vi "App - analyze RUS V6.vi"() -> ()   [LabVIEW 2018] (continued)
          tunnel: w1620 -> [w1627 w1636]
          tunnel: [w1626 w1637] -> w1619
          tunnel: [w1625 w1638] -> w1618
          tunnel: [w1624 w1640] -> w1617
          frame False {
            n725 = call <vilib>:"Color to RGB.vi"("Color"=u32 10987431) -> ("Resolved Color"=w1630:u32)  [unwired: 3 out]
            n726 = call <vilib>:"Color to RGB.vi"("Color"=u32 7500402) -> ("Resolved Color"=w1632:u32)  [unwired: 3 out]
            n727 = call <vilib>:"Color to RGB.vi"("Color"=u32 8158332) -> ("Resolved Color"=w1634:u32)  [unwired: 3 out]
            n728 = Bundle By Name(cluster=w1629, "BG Color"=w1630) -> (w1624:T43)
            n729 = Bundle By Name(cluster=w1627, "BG Color"=w1632) -> (w1626:T43)
            n730 = Bundle By Name(cluster=w1628, "BG Color"=w1634) -> (w1625:T43)
          }
          frame True {
            n731 = call <vilib>:"Color to RGB.vi"("Color"=u32 10987431) -> ("Resolved Color"=w1642:u32)  [unwired: 3 out]
            n732 = call <vilib>:"Color to RGB.vi"("Color"=u32 7500402) -> ("Resolved Color"=w1644:u32)  [unwired: 3 out]
            n733 = call <vilib>:"Color to RGB.vi"("Color"=u32 8158332) -> ("Resolved Color"=w1646:u32)  [unwired: 3 out]
            n734 = Bundle By Name(cluster=w1641, "BG Color"=w1642) -> (w1640:T43)
            n735 = Bundle By Name(cluster=w1636, "BG Color"=w1644) -> (w1637:T43)
            n736 = Bundle By Name(cluster=w1639, "BG Color"=w1646) -> (w1638:T43)
          }
        }
        n737 = property on="Tab : everything" class="TabCtl (strict)"("Colors"=w1617) -> ()  [unwired: 2 in, 2 out]
        n738 = property on="Tab :  Fit controls" class="TabCtl (strict)"("Colors"=w1618) -> ()  [unwired: 2 in, 2 out]
        n739 = property on="Tab : temperature folder" class="TabCtl (strict)"("Colors"=w1619) -> ()  [unwired: 2 in, 2 out]
      }
      event "Plot: All": Cursor Move {
        n740 = event-data() -> ("CursIdx"=w1650:i32)  [unwired: 1 in]
        n741 = case shown="3..5, Default" w1650 {
          selector: w1650 -> [w1653 w1656]
          tunnel: w1649 -> [w1652 _]
          tunnel: w1648 -> [_ w1655]
          frame 3..5, Default {
            # "zoom cursor bracket"
            n742 = call "cursor window logic V2.vi"("CursIdx"=w1653, "cursor window action"=cursor_window_action."cursor moves", "cursor window in"=w1652) -> ()  [unwired: 7 in, 2 out]
          }
          frame 0..2 {
            # "window  cursor bracket"
            n743 = call "cursor window logic V2.vi"("CursIdx"=w1656, "cursor window action"=cursor_window_action."cursor moves", "cursor window in"=w1655) -> ()  [unwired: 7 in, 2 out]
          }
        }
      }
      event User Event {
        n744 = event-data() -> ("talk to the first loop"=w1666:string)  [unwired: 1 in]
        n745 = call "slide controller.vi"("slide action"=slide_action."check", "slide control"=w1657) -> ("in slide"=w1658:bool)  [unwired: 6 in, 3 out]
        n746 = case shown="\"calculation finished\"" w1666 {
          tunnel: w1665 -> [_ _ w1688]
          tunnel: w1664 -> [_ _ w1687]
          tunnel: w1663 -> [_ w1677 _]
          tunnel: w1662 -> [_ w1675 _]
          tunnel: w1661 -> [_ w1674 _]
          tunnel: w1658 -> [_ _ w1686]
          tunnel: "plot fit progress?" -> [_ _ w1685]
          tunnel: w1657 -> [_ _ w1684]
          frame "False", Default {
          }
          frame "check fragment zoom" {
            n747 = property class="XYGraph (strict)"(reference=w1674) -> ("XScale.Maximum"=w1669:dbl, "XScale.Minimum"=w1668:dbl)  [unwired: 1 in, 2 out]
            n748 = Unbundle By Name(w1675) -> ("f (Hz)"=w1670:dbl)
            n749 = call "Q -- check range.vi"("upper"=w1669, "lower"=w1668, "number"=w1670) -> ("in range?"=w1673:bool)  [unwired: 4 in, 4 out]
            n750 = call "Q - not nan and not zero.vi"("Numeric"=w1670) -> ("Boolean"=w1671:bool)  [unwired: 10 in]
            n751 = Not(x=w1673) -> (.not. x?=w1672:bool)
            n752 = And(x=w1671, y=w1672) -> (x .and. y?=w1667:bool)
            n753 = case shown="\"when out of win\"" "zoom mode" {
              tunnel: w1677 -> [_ w1679 w1682]
              tunnel: w1667 -> [_ w1678 _]
              frame "manual", Default {
              }
              frame "when out of win" {
                n754 = case shown="False" w1678 {
                  tunnel: w1679 -> [_ w1681]
                  frame False {
                  }
                  frame True {
                    w1680 = "scale:frequency window"  # autoscale
                    n755 = Generate User Event(user event=w1681, event data cluster=w1680) -> ()  [unwired: 2 in, 2 out]
                  }
                }
              }
              frame "always" {
                w1683 = "scale:frequency window"  # autoscale
                n756 = Generate User Event(user event=w1682, event data cluster=w1683) -> ()  [unwired: 2 in, 2 out]
              }
            }
          }
          frame "calculation finished" {
            n757 = flat-sequence {
              tunnel: w1687 -> [w1694]
              tunnel: w1686 -> [w1691]
              tunnel: w1685 -> [w1693]
              tunnel: w1688 -> [w1705]
              tunnel: w1684 -> [w1698]
              frame #0 {
                n758 = Not(x=w1693) -> (.not. x?=w1692:bool)
                n759 = And(x=w1692, y=w1691) -> (x .and. y?=w1690:bool)
                n760 = Not(x=w1690) -> (.not. x?=w1689:bool)
                n761 = case shown="True" w1689 {
                  tunnel: w1694 -> [_ w1696]
                  frame False {
                  }
                  frame True {
                    (unwired) 0.0
                    n762 = Generate User Event(user event=w1696, event data cluster="redraw:all" ("event data")) -> ()  [unwired: 2 in, 2 out]
                  }
                }
              }
              frame #1 {
                w1701 = 10  # n
                # "recursively call itself while \"in slide\" is true"
                n763 = local read "in sweep folder"() -> (w1706:bool)
                n764 = call "slide controller.vi"("slide action"=slide_action."check", "slide control"=w1698) -> ("slide control OUT"=w1697:refnum<vi>, "halt event"=w1699:bool)  [unwired: 6 in, 2 out]
                n765 = And(x=w1706, y=w1699) -> (x .and. y?=w1704:bool)
                n766 = case shown="False" w1704 {
                  tunnel: w1705 -> [_ w1709]
                  tunnel: w1697 -> [w1707 _]
                  frame False {
                    n767 = call "slide controller.vi"("slide action"=slide_action."halt", "slide control"=w1707) -> ()  [unwired: 6 in, 4 out]
                  }
                  frame True {
                    w1710 = "next"  # next temperature
                    n768 = Generate User Event(user event=w1709, event data cluster=w1710) -> ()  [unwired: 2 in, 2 out]
                  }
                }
                n769 = Not(x=w1704) -> (.not. x?=w1703:bool)
                n770 = call "mean time interval.vi"("init"=w1703, "n"=w1701) -> ("mean"=→"ms/point":dbl)  [unwired: 8 in, 1 out]
              }
            }
          }
        }
      }
      event User Event {
        n771 = event-data() -> ("autoscale"=w1718:string)  [unwired: 1 in]
        n772 = local read "temperature points"() -> (w1717:dbl[])
        n773 = local read "time points"() -> (w1716:dbl[])
        n774 = case shown="\"scale:freq&atten\"" w1718 {
          tunnel: w1717 -> [_ _ _ _ w1772 _]
          tunnel: w1716 -> [_ _ _ _ _ w1773]
          tunnel: w1713 -> [w1722 _ _ _ _ _]
          tunnel: w1714 -> [w1721 _ _ _ _ _]
          tunnel: w1712 -> [_ _ w1752 _ _ _]
          tunnel: w1715 -> [w1719 _ _ _ _ _]
          tunnel: w1711 -> [_ w1747 _ _ _ _]
          frame "scale:c.plane plot zoom", Default {
            # "false- fixed\ntrue -- zoom"
            n775 = local read "c.plane scale"() -> (w1723:bool)
            n776 = Unbundle By Name(w1719) -> ("4corners.z(inf)"=w1720:cdb)
            n777 = case shown="True" w1723 {
              tunnel: w1722 -> [_ _]
              tunnel: [w1729 w1744] -> w1727
              tunnel: [w1728 w1743] -> w1726
              tunnel: [w1729 w1739] -> w1725
              tunnel: [w1728 w1738] -> w1724
              tunnel: [TRUE FALSE] -> _
              tunnel: w1721 -> [w1732 _]
              tunnel: w1720 -> [_ w1734]
              frame False {
                n778 = Unbundle By Name(w1732) -> ("pond scale factor"=w1731:dbl)
                n779 = Divide(x=w1731, y=2) -> (x/y=w1729:dbl)
                n780 = Negate(x=w1729) -> (-x=w1728:dbl)
              }
              frame True {
                w1736 = cdb 0.0+0.0i  # t
                w1740 = 0.1 ("y")
                n781 = Not A Number/Path/Refnum?(number/path/refnum=w1734) -> (NaN/Path/Refnum?=w1737:bool)
                n782 = Select(t=w1736, s=w1737, f=w1734) -> (s? t:f=w1735:cdb)
                n783 = Complex To Re/Im(x + iy=w1735) -> (x=w1742:dbl, y=w1741:dbl)
                n784 = Subtract(x=w1741, y=w1740) -> (x-y=w1738:dbl)
                n785 = Add(x=w1741, y=w1740) -> (x+y=w1739:dbl)
                n786 = Subtract(x=w1742, y=w1740) -> (x-y=w1743:dbl)
                n787 = Add(x=w1742, y=w1740) -> (x+y=w1744:dbl)
              }
            }
            n788 = property on="Plot: complex plane" class="XYGraph (strict)"("XScale.Maximum"=w1727, "XScale.Minimum"=w1726) -> ()  [unwired: 2 in, 2 out]
            n789 = property on="Plot: complex plane" class="XYGraph (strict)"("YScale.Maximum"=w1725, "YScale.Minimum"=w1724) -> ()  [unwired: 2 in, 2 out]
          }
          frame "rescale All from Zoom cursor" {
            n790 = call "cursor window logic V2.vi"("cursor window action"=cursor_window_action."zoom X", "cursor window in"=w1747) -> ()  [unwired: 8 in, 2 out]
          }
          frame "scale:frequency window" {
            n791 = Unbundle By Name(w1752) -> ("left"=w1759:dbl, "right"=w1758:dbl)
            n792 = Unbundle By Name(w1752) -> ("left"=w1755:dbl, "right"=w1754:dbl)
            n793 = Not A Number/Path/Refnum?(number/path/refnum=w1759) -> (NaN/Path/Refnum?=w1761:bool)
            n794 = Not A Number/Path/Refnum?(number/path/refnum=w1758) -> (NaN/Path/Refnum?=w1760:bool)
            n795 = Not A Number/Path/Refnum?(number/path/refnum=w1755) -> (NaN/Path/Refnum?=w1757:bool)
            n796 = Not A Number/Path/Refnum?(number/path/refnum=w1754) -> (NaN/Path/Refnum?=w1756:bool)
            n797 = Or(x=w1761, y=w1760) -> (x .or. y?=w1751:bool)
            n798 = Or(x=w1757, y=w1756) -> (x .or. y?=w1753:bool)
            n799 = Not(x=w1751) -> (.not. x?=w1750:bool)
            n800 = And(x="freq(T) : auto-adjust Y scale", y=w1750) -> (x .and. y?=w1748:bool)
            n801 = case shown="False" w1753 {
              tunnel: w1755 -> [w1764 _]
              tunnel: w1754 -> [w1763 _]
              frame False {
                n802 = local read "scale gauge: geometry plot"() -> (w1762:dbl)
                n803 = Negate(x=w1762) -> (-x=w1765:dbl)
                n804 = property on="Plot: linear map" class="XYGraph (strict)"("XScale.Minimum"=w1764, "XScale.Maximum"=w1763, "YScale.Maximum"=w1762, "YScale.Minimum"=w1765) -> ()  [unwired: 2 in, 2 out]
                n805 = property on="Plot: fragment" class="XYGraph (strict)"("XScale.Minimum"=w1764, "XScale.Maximum"=w1763) -> ()  [unwired: 2 in, 2 out]
                n806 = property on="Plot: geometry" class="XYGraph (strict)"("YScale.Maximum"=w1762, "YScale.Minimum"=w1765, "XScale.Maximum"=w1762, "XScale.Minimum"=w1765) -> ()  [unwired: 2 in, 2 out]
              }
              frame True {
              }
            }
            n807 = case shown="True" w1748 {
              tunnel: w1759 -> [_ w1767]
              tunnel: w1758 -> [_ w1766]
              frame False {
              }
              frame True {
                n808 = property on="Plot: phase around center" class="XYGraph (strict)"("XScale.Maximum"=w1766, "XScale.Minimum"=w1767) -> ()  [unwired: 2 in, 2 out]
                n809 = property on="Plot: frequency vs T" class="XYGraph (strict)"("YScale.Maximum"=w1766, "YScale.Minimum"=w1767) -> ()  [unwired: 2 in, 2 out]
              }
            }
          }
          frame "scale:freq&atten" {
            n810 = property on="Plot: delta f" class="XYGraph (strict)"() -> ("XScale.Maximum"=w1768:dbl, "XScale.Minimum"=w1769:dbl)  [unwired: 2 in, 2 out]
            n811 = property on="Plot: frequency vs T" class="XYGraph (strict)"("XScale.Maximum"=w1768, "XScale.Minimum"=w1769) -> ()  [unwired: 2 in, 2 out]
            n812 = property on="Plot: attenuation vs T" class="XYGraph (strict)"("XScale.Maximum"=w1768, "XScale.Minimum"=w1769) -> ()  [unwired: 2 in, 2 out]
          }
          frame "scale:temperature" {
            n813 = Array Max & Min(array=w1772) -> (max value=w1771:dbl, min value=w1770:dbl)  [unwired: 2 out]
            n814 = property on="Plot: delta f" class="XYGraph (strict)"("XScale.Maximum"=w1771, "XScale.Minimum"=w1770) -> ()  [unwired: 2 in, 2 out]
            n815 = property on="Plot: frequency vs T" class="XYGraph (strict)"("XScale.Maximum"=w1771, "XScale.Minimum"=w1770) -> ()  [unwired: 2 in, 2 out]
            n816 = property on="Plot: attenuation vs T" class="XYGraph (strict)"("XScale.Maximum"=w1771, "XScale.Minimum"=w1770) -> ()  [unwired: 2 in, 2 out]
          }
          frame "scale:position" {
            n817 = Array Size(array=w1773) -> (size(s)=w1776:i32)
            n818 = Decrement(x=w1776) -> (x-1=w1777:i32)
            n819 = Index Array(array=w1773, index=w1777) -> (element=w1778:dbl)
            n820 = Index Array(array=w1773, index=0) -> (element=w1779:dbl)
            n821 = Max & Min(x=w1778, y=w1779) -> (max(x,y)=w1774:dbl, min(x,y)=w1788:dbl)
            n822 = Add(x=w1788, y=w1774) -> (x+y=w1783:dbl)
            n823 = property on="Plot: Time" class="XYGraph (strict)"("XScale.Maximum"=w1774, "XScale.Minimum"=w1788) -> ()  [unwired: 2 in, 2 out]
            n824 = Divide(x=w1783, y=2.0) -> (x/y=w1785:dbl)
            n825 = property on="Plot: Time" class="XYGraph (strict)"() -> ("CrsrList"=w1780:T44)  [unwired: 2 in, 2 out]
            n826 = call "replace cursor.vi"("action"=enum16{"", "read", "write"}."write" ("Enum"), "cursor index"=0, "new  Y"=0.0, "new X"=w1785, "Cursor List in"=w1780) -> ("Cursor List Out"=w1787:T44)  [unwired: 4 in, 2 out]
            n827 = property on="Plot: Time" class="XYGraph (strict)"("CrsrList"=w1787) -> ()  [unwired: 2 in, 2 out]
          }
        }
      }
      event User Event {
        n828 = event-data() -> ("show plot pallets"=w1789:bool)  [unwired: 1 in]
        n829 = property on="Plot: phase around center" class="XYGraph (strict)"("ScaleLegendVis"=w1789, "Palette Visible"=w1789, "Legend Visible"=w1789) -> ()  [unwired: 2 in, 2 out]
        n830 = property on="Plot: fragment" class="XYGraph (strict)"("ScaleLegendVis"=w1789, "Palette Visible"=w1789, "Legend Visible"=w1789) -> ()  [unwired: 2 in, 2 out]
        n831 = property on="Plot: frequency vs T" class="XYGraph (strict)"("ScaleLegendVis"=w1789, "Palette Visible"=w1789, "Legend Visible"=w1789) -> ()  [unwired: 2 in, 2 out]
        n832 = property on="Plot: attenuation vs T" class="XYGraph (strict)"("ScaleLegendVis"=w1789, "Palette Visible"=w1789, "Legend Visible"=w1789) -> ()  [unwired: 2 in, 2 out]
        n833 = property on="Plot: delta f" class="XYGraph (strict)"("ScaleLegendVis"=w1789, "Palette Visible"=w1789, "Legend Visible"=w1789) -> ()  [unwired: 2 in, 2 out]
        n834 = property on="Plot: All" class="XYGraph (strict)"("ScaleLegendVis"=w1789, "Palette Visible"=w1789, "Legend Visible"=w1789) -> ()  [unwired: 2 in, 2 out]
        n835 = property on="Plot: geometry" class="XYGraph (strict)"("ScaleLegendVis"=w1789, "Palette Visible"=w1789, "Legend Visible"=w1789) -> ()  [unwired: 2 in, 2 out]
        n836 = property on="Plot: linear map" class="XYGraph (strict)"("ScaleLegendVis"=w1789, "Palette Visible"=w1789, "Legend Visible"=w1789) -> ()  [unwired: 2 in, 2 out]
        n837 = property on="Plot: Time" class="XYGraph (strict)"("ScaleLegendVis"=w1789, "Palette Visible"=w1789, "Legend Visible"=w1789) -> ()  [unwired: 2 in, 2 out]
      }
      event User Event {
        n838 = event-data() -> ("redraw"=w1826:string)  [unwired: 1 in]
        n839 = local read "temperature points"() -> (w1823:dbl[])
        n840 = local read "frequency points"() -> (w1825:dbl[])
        n841 = local read "attenuation points"() -> (w1824:dbl[])
        n842 = local read "time points"() -> (w1820:dbl[])
        n843 = local read "time (min)"() -> (w1822:dbl)
        n844 = local read "Magn Field points"() -> (w1792:dbl[])
        n845 = local read "phase points"() -> (w1821:dbl[])
        n846 = local read "power points"() -> (w1794:dbl[])
        n847 = local read "ampl points"() -> (w1804:dbl[])
        n848 = control-ref of="Plot: complex plane"() -> (w1812:refnum<vi>)
        n849 = local read "fit using"() -> (w1806:T5)
        n850 = call "slide controller.vi"("slide action"=slide_action."check", "slide control"=w1798) -> ("in slide"=w1799:bool)  [unwired: 6 in, 3 out]
        n851 = case shown="\"redraw:freq/atten\"" w1826 {
          selector: w1826 -> [_ _ _ _ _ _ w1979 _ _ _]
          tunnel: w1827 -> [_ _ _ w1918 w1929 _ _ _ _ _]
          tunnel: w1816 -> [_ w1890 _ _ _ _ _ _ _ _]
          tunnel: w1817 -> [_ _ _ _ _ _ w1978 w2048 w2058 w2075]
          tunnel: w1814 -> [_ _ _ w1920 _ _ _ _ _ _]
          tunnel: w1818 -> [_ w1885 _ _ _ w1951 _ _ _ _]
          tunnel: w1815 -> [_ w1888 _ _ _ _ _ _ _ _]
          tunnel: w1813 -> [_ w1887 _ _ _ _ _ _ _ _]
          tunnel: w1819 -> [_ w1886 _ _ _ w1950 _ _ _ _]
          tunnel: w1825 -> [_ _ _ _ _ _ w1977 _ w2068 w2076]
          tunnel: w1824 -> [_ _ _ _ _ _ w1976 _ _ w2071]
          tunnel: w1823 -> [_ _ _ _ _ _ w1975 w2032 w2062 _]
          tunnel: w1822 -> [_ _ _ _ _ _ w1974 w2047 _ _]
          tunnel: w1821 -> [_ _ _ _ _ _ w1973 _ _ _]
          tunnel: w1820 -> [_ _ _ _ _ _ w1972 w2029 _ _]
          tunnel: w1809 -> [_ _ _ _ _ _ w1971 _ _ _]
          tunnel: w1793 -> [_ _ _ _ _ _ w1970 _ _ _]
          tunnel: w1812 -> [_ w1884 _ _ _ _ _ _ _ _]
          tunnel: "plot when in slide" -> [_ _ _ _ _ _ w1967 _ _ _]
          tunnel: w1799 -> [_ _ _ _ _ _ w1965 _ _ _]
          tunnel: w1810 -> [_ _ _ _ _ _ w1963 _ w2061 _]
          tunnel: w1808 -> [_ _ _ _ _ _ w1962 _ _ _]
          tunnel: w1807 -> [_ _ _ _ _ _ w1961 _ w2060 _]
          tunnel: w1806 -> [_ _ _ _ _ _ w1960 _ _ _]
          tunnel: w1805 -> [_ _ _ _ _ _ w1959 w2039 _ _]
          tunnel: w1804 -> [_ _ _ _ _ _ w1958 _ _ _]
          tunnel: w1803 -> [_ _ _ _ _ _ w1957 _ _ _]
          tunnel: w1802 -> [_ _ _ _ _ _ w1956 _ _ _]
          tunnel: w1801 -> [_ _ _ _ _ w1936 _ _ _ _]
          tunnel: w1797 -> [_ _ _ _ _ _ w1955 _ _ _]
          tunnel: w1796 -> [_ _ _ _ _ _ w1954 _ _ _]
          tunnel: w1795 -> [_ _ _ _ _ _ w1953 _ _ _]
          tunnel: w1794 -> [_ _ _ _ _ _ w1952 _ _ _]
          tunnel: w1792 -> [_ _ _ _ _ _ _ w2028 _ w2072]
          tunnel: w1791 -> [_ _ _ _ _ _ _ _ _ w2070]
          tunnel: w1790 -> [_ _ _ _ _ _ _ _ _ w2069]
          frame "False", Default {
          }
          frame "redraw:fit related" {
            w1841 = 0.5
            (unwired) FALSE
            # "cursor 1 follows z(inf)\ncursor  2 follows z(0)"
            n852 = Unbundle By Name(w1886) -> ("4corners"=w1889:T12)
            n853 = Unbundle By Name(w1885) -> ("omega in window"=w1865:dbl[], "phase around center"=w1872:dbl[], "three points"=w1863:cluster{dbl[], dbl[]}, "inverse"=w1876:cdb[], "linear"=w1875:cdb[], "omega around"=w1874:dbl[])
            n854 = Unbundle By Name(w1889) -> ("z center"=w1830:cdb, "z(inf)"=w1831:cdb)
            n855 = Unbundle By Name(w1885) -> ("normalized z"=w1835:cdb[], "number of 2D grid points"=w1828:i32)
            n856 = Unbundle By Name(w1888) -> ("wave number"=w1837:dbl)
            n857 = Unbundle By Name(w1889) -> ("z center"=w1829:cdb, "z(0)"=w1844:cdb)
            n858 = Unbundle By Name(w1887) -> ("delta  z"=w1838:cdb)
            n859 = Unbundle By Name(w1890) -> ("omega"=w1869:dbl, "gamma"=w1868:dbl, "theta0"=w1867:dbl)
            n860 = Build Array(w1869, w1868, w1867) -> (w1866:dbl[])
            n861 = Complex To Re/Im(x + iy=w1838) -> (x=w1839:dbl)  [unwired: 1 out]
            n862 = Complex To Re/Im(x + iy=w1831) -> (x=w1857:dbl, y=w1856:dbl)
            n863 = flat-sequence {
              tunnel: w1886 -> [w1910]
              tunnel: w1889 -> [w1909]
              tunnel: w1874 -> [w1898]
              tunnel: [w1897] -> w1873
              frame #0 {
                n864 = Unbundle By Name(w1909) -> ("z center"=w1908:cdb, "z(inf)"=w1906:cdb)
                n865 = Unbundle By Name(w1910) -> ("f (Hz)"=w1904:dbl, "G (Hz)"=w1902:dbl)
                n866 = Subtract(x=w1908, y=w1906) -> (x-y=w1907:cdb)
                n867 = Subtract(x=w1898, y=w1904) -> (x-y=w1903:dbl[])
                n868 = Multiply(x=w1907, y=cdb 2.0+0.0i) -> (x*y=w1894:cdb)
                n869 = Multiply(x=cdb 0.0-1.0i ("y"), y=w1894) -> ()  [unwired: 1 out]
                n870 = Divide(x=w1903, y=w1902) -> (x/y=w1901:dbl[])
                n871 = Add(x=w1894, y=w1906) -> ()  [unwired: 1 out]
                n872 = Multiply(x=w1901, y=2) -> (x*y=w1899:dbl[])
                n873 = Complex To Polar(r * e^(i*theta)=w1894) -> (r=w1893:dbl)  [unwired: 1 out]
                n874 = Negate(x=w1893) -> (-x=w1892:dbl)
                n875 = Multiply(x=w1899, y=w1892) -> (x*y=w1895:dbl[])
                n876 = Bundle("omega around"=w1898, w1895) -> (w1897:cluster{"omega around":dbl[], dbl[]})  [unwired: 1 in]
              }
            }
            n877 = call "omega map fit function.vi"("X"=w1865, "a"=w1866) -> ("f(X,a)"=w1864:dbl[])  [unwired: 2 in, 2 out]
            n878 = call "replace cursor - plot ref.vi"("action"=enum16{"", "read", "write"}."write" ("Enum"), "cursor index"=1, "new  Y"=w1856, "new X"=w1857, "Plot ref in"=w1884) -> ("Plot ref out"=w1836:refnum<vi>)  [unwired: 4 in, 2 out]
            n879 = Divide(x=w1839, y=w1828) -> (x/y=w1840:dbl)
            n880 = Complex To Re/Im(x + iy=w1835) -> (x=w1861:dbl[], y=w1860:dbl[])
            n881 = Divide(x=w1839, y=w1837) -> (x/y=w1849:dbl)
            n882 = Complex To Re/Im(x + iy=w1830) -> (x=w1853:dbl, y=w1852:dbl)
            n883 = Add(x=w1849, y=w1840) -> (x+y=w1848:dbl)
            n884 = Complex To Re/Im(x + iy=w1829) -> (x=w1845:dbl, y=w1846:dbl)
            n885 = Subtract(x=w1844, y=w1829) -> (x-y=w1843:cdb)
            n886 = Bundle("omega in window"=w1865, "f(X,a)"=w1864) -> (w1862:cluster{"omega in window":dbl[], "f(X,a)":dbl[]})  [unwired: 1 in]
            n887 = Bundle("omega in window"=w1865, "phase around center"=w1872) -> (w1871:T45)  [unwired: 1 in]
            n888 = Bundle(w1861, w1860) -> (w1891:cluster{dbl[], dbl[]})  [unwired: 1 in]
            n889 = Complex To Polar(r * e^(i*theta)=w1843) -> (theta=w1842:dbl)  [unwired: 1 out]
            n890 = call "replace cursor - plot ref.vi"("action"=enum16{"", "read", "write"}."write" ("Enum"), "cursor index"=2, "new  Y"=w1852, "new X"=w1853, "Plot ref in"=w1836) -> ()  [unwired: 4 in, 3 out]
            n891 = Build Array(w1871, w1863, w1862) -> (→"Plot: phase around center":T46)
            n892 = call "draw a circle.vi"("angular arc bounds"=w1841, "angular arc center"=w1842, "center Y"=w1846, "center x"=w1845, "radius"=w1849) -> ("output cluster"=w1850:cluster{dbl[], dbl[]})  [unwired: 6 in]
            n893 = call "draw a circle.vi"("angular arc bounds"=w1841, "angular arc center"=w1842, "center Y"=w1846, "center x"=w1845, "radius"=w1848) -> ("output cluster"=w1847:cluster{dbl[], dbl[]})  [unwired: 6 in]
            n894 = Complex To Re/Im(x + iy=w1875) -> (x=w1879:dbl[])  [unwired: 1 out]
            n895 = Complex To Re/Im(x + iy=w1876) -> (x=w1882:dbl[], y=w1881:dbl[])
            n896 = call "draw - 4 corner circle.vi"("4corners"=w1889) -> ("line two"=w1832:cluster{dbl[], dbl[]}, "line one"=w1833:cluster{dbl[], dbl[]}, "circle"=w1834:cluster{dbl[], dbl[]})  [unwired: 8 in]
            n897 = Bundle(w1882, w1881) -> (w1880:cluster{dbl[], dbl[]})  [unwired: 1 in]
            n898 = Bundle("omega around"=w1874, w1879) -> (w1878:cluster{"omega around":dbl[], dbl[]})  [unwired: 1 in]
            n899 = Build Array(w1891, w1880) -> (→"Plot: geometry":cluster{dbl[], dbl[]}[])
            n900 = Build Array(w1891, w1834, w1833, w1832, w1850, w1847) -> (→"Plot: complex plane":cluster{dbl[], dbl[]}[])
            n901 = Build Array(w1878, w1873) -> (→"Plot: linear map":cluster{"omega around":dbl[], dbl[]}[])
          }
          frame "plot filter progress" {
            n902 = control-ref of="Tab : fit/filter progress"() -> (w1916:refnum<vi>)
            n903 = local read "plot filter progress?"() -> (w1912:bool)
            n904 = Not(x=w1912) -> (.not. x?=w1911:bool)
            n905 = Select(t=enum32{"Page 1", "Page 2"}."Page 2" ("Value"), s=w1911, f=enum32{"Page 1", "Page 2"}."Page 1" ("Value")) -> (s? t:f=w1915:enum32{"Page 1", "Page 2"})
            n906 = property class="TabCtl (strict)"(reference=w1916, "Value"=w1915) -> ()  [unwired: 1 in, 2 out]
            n907 = local write "plot filter progress?"(w1911) -> ()
          }
          frame "redraw:all" {
            n908 = case shown="True" "old staff plot" {
              tunnel: [w1921 w1923] -> w1919
              tunnel: w1918 -> [w1921 w1922]
              frame False {
              }
              frame True {
                n909 = Generate User Event(user event=w1922, event data cluster="redraw:fit and fragment" ("event data")) -> (user event out=w1923:refnum<user-event>)  [unwired: 2 in, 1 out]
              }
            }
            n910 = case shown="True" w1920 {
              tunnel: w1919 -> [_ w1927]
              frame False {
              }
              frame True {
                n911 = Generate User Event(user event=w1927, event data cluster="redraw:freq/atten" ("event data")) -> (user event out=w1926:refnum<user-event>)  [unwired: 2 in, 1 out]
                n912 = Generate User Event(user event=w1926, event data cluster="redraw:magn field" ("event data")) -> ()  [unwired: 2 in, 2 out]
              }
            }
          }
          frame "redraw:fit and fragment" {
            n913 = Generate User Event(user event=w1929, event data cluster="redraw:fragment" ("event data")) -> (user event out=w1932:refnum<user-event>)  [unwired: 2 in, 1 out]
            n914 = Generate User Event(user event=w1932, event data cluster="redraw:fit related" ("event data")) -> ()  [unwired: 2 in, 2 out]
          }
          frame "redraw:fragment" {
            # "construct Lorentzian"
            n915 = Unbundle By Name(w1951) -> ("omega in window"=w1949:dbl[], "normalized z"=w1948:cdb[])
            n916 = disable-structure shown="Disabled" {
              frame Disabled {
                n917 = local read item#-1() -> ()  [unwired: 1 out]
                n918 = local read item#-1() -> ()  [unwired: 1 out]
              }
              frame Enabled {
              }
            }
            n919 = Unbundle By Name(w1950) -> ("f (Hz)"=w1935:dbl)
            n920 = call "replace cursor - plot ref.vi"("action"=enum16{"", "read", "write"}."write", "cursor index"=3, "new X"=w1935, "Plot ref in"=w1936) -> ()  [unwired: 5 in, 3 out]
            n921 = call "construct lorentzian.vi"("omega  in"=w1949, "lorentzian"=w1950) -> ("omega  out"=w1940:dbl[], "z out"=w1941:cdb[])  [unwired: 8 in]
            n922 = Complex To Re/Im(x + iy=w1948) -> (x=w1945:dbl[], y=w1944:dbl[])
            n923 = Complex To Re/Im(x + iy=w1941) -> (x=w1943:dbl[], y=w1942:dbl[])
            n924 = Bundle("omega in window"=w1949, w1945) -> (w1939:cluster{"omega in window":dbl[], dbl[]})  [unwired: 1 in]
            n925 = Bundle("omega  out"=w1940, w1943) -> (w1947:cluster{"omega  out":dbl[], dbl[]})  [unwired: 1 in]
            n926 = Bundle("omega  out"=w1940, w1942) -> (w1946:cluster{"omega  out":dbl[], dbl[]})  [unwired: 1 in]
            n927 = Bundle("omega in window"=w1949, w1944) -> (w1938:cluster{"omega in window":dbl[], dbl[]})  [unwired: 1 in]
            n928 = Build Array(w1939, w1938, w1947, w1946) -> (→"Plot: fragment":cluster{"omega  out":dbl[], dbl[]}[])
          }
          frame "redraw:freq/atten" {
            n929 = call "counter-i.vi"("init ?"=w1956, "cricket interval"=30 ("interval")) -> ("cricket"=w1968:bool)  [unwired: 8 in, 1 out]
            n930 = Not(x=w1965) -> (.not. x?=w1964:bool)
            n931 = Compound Arithmetic op=OR(w1967, w1968, w1964) -> (w1966:bool)
            n932 = case shown="True" w1966 {
              tunnel: w1979 -> [_ w2000]
              tunnel: w1978 -> [_ w1999]
              tunnel: w1977 -> [_ w1998]
              tunnel: w1976 -> [_ w1997]
              tunnel: w1975 -> [_ w1996]
              tunnel: w1974 -> [_ w1995]
              tunnel: w1973 -> [_ w1994]
              tunnel: w1972 -> [_ w1993]
              tunnel: w1971 -> [_ w1987]
              tunnel: w1970 -> [_ w1992]
              tunnel: w1963 -> [_ w1991]
              tunnel: w1962 -> [_ w1990]
              tunnel: w1961 -> [_ w1989]
              tunnel: w1960 -> [_ w1988]
              tunnel: w1959 -> [_ w1986]
              tunnel: w1958 -> [_ w1985]
              tunnel: w1957 -> [_ w1984]
              tunnel: w1955 -> [_ w1983]
              tunnel: w1954 -> [_ w1982]
              tunnel: w1953 -> [_ w1981]
              tunnel: w1952 -> [_ w1980]
              frame False {
              }
              frame True {
                n933 = flat-sequence {
                  tunnel: w2000 -> [_]
                  tunnel: [w2026] -> _
                  tunnel: w1999 -> [w2010]
                  tunnel: w1998 -> [w2004]
                  tunnel: w1997 -> [w2003]
                  tunnel: w1996 -> [w2013]
                  tunnel: w1995 -> [w2025]
                  tunnel: w1994 -> [_]
                  tunnel: w1993 -> [w2018]
                  tunnel: w1987 -> [w2019]
                  tunnel: w1992 -> [w2024]
                  tunnel: w1991 -> [_]
                  tunnel: w1990 -> [w2021]
                  tunnel: w1989 -> [w2020]
                  tunnel: w1988 -> [w2016]
                  tunnel: w1986 -> [_]
                  tunnel: [w2019] -> _
                  tunnel: w1985 -> [_]
                  tunnel: w1984 -> [_]
                  tunnel: w1983 -> [w2012]
                  tunnel: w1982 -> [w2006]
                  tunnel: w1981 -> [w2005]
                  tunnel: w1980 -> [w2002]
                  frame #0 {
                    w2007 = T3."linear-linear" ("mapping")
                    (unwired) FALSE  # plot phase/ampl
                    (unwired) TRUE
                    # "\"scale:frequency window\""
                    # "current point"
                    n934 = Generate User Event(user event=w2012, event data cluster="scale:freq&atten" ("event data")) -> ()  [unwired: 2 in, 2 out]
                    n935 = call "fit function selector.vi"("fit using"=w2016, "temperature"=w2013) -> ("freq out"=w2014:dbl[])  [unwired: 7 in, 2 out]
                    n936 = Subtract(x=w2004, y=w2014) -> (x-y=w2017:dbl[])
                    "delta-f points" <- w2017
                    n937 = Threshold 1D Array(2:w2025, 3:w2018) -> (0:w2027:dbl)  [unwired: 1 in]
                    n938 = Index Array(array=w2013, index=w2027) -> (element=w2026:dbl)
                    n939 = call "color split.vi"("point style"=enum16{"dot", "cross"}."dot", "mapping"=w2020, "tfolder"=w2010, "Plot Ref"=w2019, "Y"=w2004, "X"=w2013) -> ()  [unwired: 5 in, 1 out]
                    n940 = call "color split.vi"("point style"=enum16{"dot", "cross"}."dot", "mapping"=w2020, "tfolder"=w2010, "Plot Ref"=w2024, "Y"=w2003, "X"=w2013) -> ()  [unwired: 5 in, 1 out]
                    n941 = call "color split.vi"("point style"=enum16{"dot", "cross"}."dot", "mapping"=w2007, "tfolder"=w2010, "Plot Ref"=w2005, "Y"=w2003, "X"=w2002) -> ()  [unwired: 5 in, 1 out]
                    n942 = call "color split.vi"("point style"=enum16{"dot", "cross"}."dot", "mapping"=w2007, "tfolder"=w2010, "Plot Ref"=w2006, "Y"=w2004, "X"=w2002) -> ()  [unwired: 5 in, 1 out]
                    n943 = call "color split.vi"("point style"=enum16{"dot", "cross"}."dot", "mapping"="mapping delta f vs T", "tfolder"=w2010, "Plot Ref"=w2021, "Y"=w2017, "X"=w2013) -> ()  [unwired: 5 in, 1 out]
                  }
                }
              }
            }
          }
          frame "redraw:time" {
            w2036 = FALSE  # Name Visible
            # "current point"
            n944 = Threshold 1D Array(2:w2047, 3:w2029) -> (0:w2046:dbl)  [unwired: 1 in]
            n945 = Index Array(array=w2032, index=w2046) -> (element=w2041:dbl)
            n946 = Index Array(array=w2029, index=w2046) -> (element=w2043:dbl)
            n947 = Build Array(w2043) -> (w2042:dbl[])
            n948 = Build Array(w2041) -> (w2044:dbl[])
            n949 = Bundle(w2042, w2044) -> (w2045:cluster{dbl[], dbl[]})  [unwired: 1 in]
            n950 = Bundle("time points"=w2029, "temperature points"=w2032) -> (w2051:T47)  [unwired: 1 in]
            n951 = Build Array(w2045, w2051) -> (w2040:T48)
            n952 = Array Size(array=w2040) -> (size(s)=w2037:i32)
            n953 = call "derivative.vi"("temperature (min)"=w2029, "frequency (kHz)"=w2032) -> ("derivative (kHz/min)"=w2033:dbl[])  [unwired: 9 in]
            n954 = for {
              N: w2037 -> [_]
              tunnel: w2039 -> [w2057]
              tunnel: [w2056] -> w2038
              i -> [w2055]
              n955 = call "plot -- make visible.vi"("Active Plot"=w2055, "reference"=w2057) -> ("reference out"=w2056:refnum<vi>)  [unwired: 9 in]
            }
            n956 = Bundle("temperature points"=w2032, "derivative (kHz/min)"=w2033) -> (w2035:T49)  [unwired: 1 in]
            n957 = Bundle("time points"=w2029, "Magn Field points"=w2028) -> (w2031:T50)  [unwired: 1 in]
            n958 = call "color split.vi"("point style"=enum16{"dot", "cross"}."cross", "tfolder"=w2048, "Plot Ref"=w2038, "plot array IN"=w2040, "Y"=w2032, "X"=w2029) -> ("plot array OUT"=w2050:T51)  [unwired: 5 in]
            n959 = Build Array(w2035) -> (→"Plot: dTemp/dTime":T52)
            n960 = Build Array(w2031) -> (w2030:T53)
            n961 = Unbundle By Name(w2048) -> ("timestamp array"=w2054:dbl[])
            n962 = local write "Plot: H vs Time"(w2030) -> ()
            n963 = Array Max & Min(array=w2032) -> (max value=w2053:dbl, min value=w2052:dbl)  [unwired: 2 out]
            n964 = call "generate comb.vi"("maxY"=w2053, "Name Visible"=w2036, "minY"=w2052, "Plot Ref"=w2038, "freq array"=w2054, "plot list IN"=w2050) -> ()  [unwired: 5 in, 1 out]
          }
          frame "redraw:dfdt" {
            w2059 = enum16{"dot", "cross"}."dot"  # point style
            n965 = call "derivative d Log f.vi"("log T ?"="log T ?", "requested size"="derivative window", "temperature (min)"=w2062, "frequency (kHz)"=w2068) -> ("derivative (kHz/min)"=w2067:dbl[])  [unwired: 7 in]
            n966 = Multiply(x=w2067, y="zoom factor - derivative") -> (x*y=w2063:dbl[])
            n967 = call "color split.vi"("point style"=w2059, "mapping"=w2060, "tfolder"=w2058, "Plot Ref"=w2061, "Y"=w2063, "X"=w2062) -> ()  [unwired: 5 in, 1 out]
          }
          frame "redraw:magn field" {
            w2073 = T3."linear-linear" ("mapping")
            w2074 = enum16{"dot", "cross"}."dot"  # point style
            n968 = call "color split.vi"("point style"=w2074, "mapping"=w2073, "tfolder"=w2075, "Plot Ref"=w2070, "Y"=w2076, "X"=w2072) -> ()  [unwired: 5 in, 1 out]
            n969 = call "color split.vi"("point style"=w2074, "mapping"=w2073, "tfolder"=w2075, "Plot Ref"=w2069, "Y"=w2071, "X"=w2072) -> ()  [unwired: 5 in, 1 out]
          }
        }
      }
      event User Event {
        n970 = event-data() -> ("cursors"=w2083:string)  [unwired: 1 in]
        n971 = case shown="\"cursors:init all\", Default" w2083 {
          tunnel: cursor_window_action."check" ("cursor window action") -> [_ _ w2137]
          tunnel: w2078 -> [w2085 _ _]
          tunnel: w2079 -> [w2084 _ _]
          tunnel: w2081 -> [w2089 _ w2140]
          tunnel: w2080 -> [w2088 _ w2139]
          tunnel: w2082 -> [w2087 _ w2138]
          frame "cursors:init all", Default {
            w2086 = cursor_window_action."init" ("cursor window action")
            # "init satff"
            n972 = local read "cursor bracket: All, data window"() -> (w2096:T24)
            n973 = Build Array(0, 1, 2) -> (w2106:i32[])
            n974 = local read "cursor bracket: All,  zoom"() -> (w2102:T24)
            n975 = Build Array(3, 4, 5) -> (w2101:i32[])
            n976 = Build Array(0, 1, 2) -> (w2100:i32[])
            n977 = local read "cursor bracket: fragment"() -> (w2098:T24)
            n978 = Bundle By Name(cluster=w2098, "Plot ref"=w2085, "cursors"=w2100) -> (w2099:T24)
            n979 = Bundle By Name(cluster=w2102, "Plot ref"=w2084, "cursors"=w2101) -> (w2103:T24)
            n980 = Bundle By Name(cluster=w2096, "Plot ref"=w2084, "cursors"=w2106) -> (w2097:T24)
            n981 = call "cursor window logic V2.vi"("cursor window action"=w2086, "cursor window in"=w2087, "cursor window init"=w2099) -> ()  [unwired: 7 in, 2 out]
            n982 = call "cursor window logic V2.vi"("cursor window action"=w2086, "cursor window in"=w2088, "cursor window init"=w2103) -> ()  [unwired: 7 in, 2 out]
            n983 = call "cursor window logic V2.vi"("cursor window action"=w2086, "cursor window in"=w2089, "cursor window init"=w2097) -> ()  [unwired: 7 in, 2 out]
          }
          frame "cursor:init colors" {
            w2114 = "zoom:right"  # Name
            w2116 = "zoom:center"  # Name
            w2117 = "zoom:left"  # Name
            w2122 = "win:right"  # Name
            w2124 = "win:center"  # Name
            w2125 = "win:left"  # Name
            w2128 = 0  # index
            w2130 = "win:left"  # Name
            w2136 = u32 0  # Cursor Mode
            w2135 = TRUE  # Allow Drag
            w2134 = FALSE  # Name Visible
            w2133 = u8 0  # Point Style
            w2132 = u8 2  # Style
            w2129 = T44 [{"Name"="win:left", "Color"=16771584, "Style"=2, "Point Style"=0, "Name Visible"=FALSE, "Allow Drag"=TRUE, "Cursor Mode"=0, "Plot"=0, "Index"=0, "Position"={"X"=2535.2200767392833, "Y"=0.0}, "X Scale"=0, "Y Scale"=0, "Watch Plots"=[], "Watch All Plots"=FALSE, "Plot Area"=0, "Label Offset"={"X"=0.6062171324215342, "Y"=9.61538461538465e-05}}, {"Name"="win:center", "Color"=16776960, "Style"=2, "Point Style"=0, "Name Visible"=FALSE, "Allow Drag"=TRUE, "Cursor Mode"=0, "Plot"=0, "Index"=0, "Position"={"X"=2557.3470020726513, "Y"=0.0}, "X Scale"=0, "Y Scale"=0, "Watch Plots"=[], "Watch All Plots"=FALSE, "Plot Area"=0, "Label Offset"={"X"=0.3031085662105397, "Y"=9.61538461538465e-05}}, {"Name"="win:right", "Color"=16771584, "Style"=2, "Point Style"=0, "Name Visible"=FALSE, "Allow Drag"=TRUE, "Cursor Mode"=0, "Plot"=0, "Index"=0, "Position"={"X"=2579.4739274060194, "Y"=0.0}, "X Scale"=0, "Y Scale"=0, "Watch Plots"=[], "Watch All Plots"=FALSE, "Plot Area"=0, "Label Offset"={"X"=0.6062171324210794, "Y"=9.61538461538465e-05}}, {"Name"="zoom:left", "Color"=9013641, "Style"=2, "Point Style"=6, "Name Visible"=FALSE, "Allow Drag"=TRUE, "Cursor Mode"=0, "Plot"=0, "Index"=0, "Position"={"X"=2438.615046565618, "Y"=0.0}, "X Scale"=0, "Y Scale"=0, "Watch Plots"=[], "Watch All Plots"=FALSE, "Plot Area"=0, "Label Offset"={"X"=-0.08660244748853074, "Y"=9.61538461538465e-05}}, {"Name"="zoom:center", "Color"=9013641, "Style"=2, "Point Style"=6, "Name Visible"=FALSE, "Allow Drag"=TRUE, "Cursor Mode"=0, "Plot"=0, "Index"=0, "Position"={"X"=2518.3975513146, "Y"=0.0}, "X Scale"=0, "Y Scale"=0, "Watch Plots"=[], "Watch All Plots"=FALSE, "Plot Area"=0, "Label Offset"={"X"=0.15155428310526986, "Y"=9.61538461538465e-05}}, {"Name"="zoom:right", "Color"=9013641, "Style"=2, "Point Style"=6, "Name Visible"=FALSE, "Allow Drag"=TRUE, "Cursor Mode"=0, "Plot"=0, "Index"=0, "Position"={"X"=2598.1800560635825, "Y"=0.0}, "X Scale"=0, "Y Scale"=0, "Watch Plots"=[], "Watch All Plots"=FALSE, "Plot Area"=0, "Label Offset"={"X"=0.08660244748853074, "Y"=9.61538461538465e-05}}]  # all cursor list
            # "setup cursors"
            n984 = Index Array(array=w2129, index=w2128) -> (element=w2127:T54)
            n985 = Bundle By Name(cluster=w2127, "Name"=w2130, "Color"=u32 16768256, "Style"=w2132, "Point Style"=w2133, "Name Visible"=w2134, "Allow Drag"=w2135, "Cursor Mode"=w2136) -> (w2110:T54)
            n986 = Bundle By Name(cluster=w2110, "Name"=w2117, "Color"=u32 7763574) -> (w2113:T54)
            n987 = Bundle By Name(cluster=w2110, "Name"=w2125, "Color"=u32 13696834) -> (w2121:T54)
            n988 = Bundle By Name(cluster=w2110, "Name"=w2116, "Color"=u32 13816530) -> (w2112:T54)
            n989 = Bundle By Name(cluster=w2110, "Name"=w2114, "Color"=u32 10132122) -> (w2111:T54)
            n990 = Bundle By Name(cluster=w2110, "Name"=w2124, "Color"=u32 16252785) -> (w2120:T54)
            n991 = Bundle By Name(cluster=w2110, "Name"=w2122, "Color"=u32 13959025) -> (w2119:T54)
            n992 = Build Array(w2113, w2112, w2111) -> ()  [unwired: 1 out]
            n993 = Build Array(w2121, w2120, w2119) -> ()  [unwired: 1 out]
          }
          frame "cursors:check all" {
            n994 = call "cursor window logic V2.vi"("cursor window action"=w2137, "cursor window in"=w2138) -> ()  [unwired: 8 in, 2 out]
            n995 = call "cursor window logic V2.vi"("cursor window action"=w2137, "cursor window in"=w2139) -> ()  [unwired: 8 in, 2 out]
            n996 = call "cursor window logic V2.vi"("cursor window action"=w2137, "cursor window in"=w2140) -> ()  [unwired: 8 in, 2 out]
          }
        }
      }
      event "scale gauge: geometry plot": Value Change {
        (unwired) FALSE ("event data")
        n997 = event-data() -> ()  [unwired: 1 in, 1 out]
        n998 = Generate User Event(user event=w2141, event data cluster="scale:frequency window" ("event data")) -> ()  [unwired: 2 in, 2 out]
      }
      event "Plot: Time": Cursor Move {
        n999 = event-data() -> ("CursIdx"=w2145:i32)  [unwired: 1 in]
        n1000 = case shown="1..3" w2145 {
          selector: w2145 -> [w2147 w2159]
          tunnel: w2144 -> [_ w2158]
          tunnel: w2143 -> [w2149 _]
          frame 0, Default {
            w2150 = enum16{"hide", "show x", "show y", "show (x,y)"}."hide"  # label
            w2154 = enum16{"", "read", "write"}."write"  # action
            w2156 = enum16{"", "read", "write"}."read"  # action
            # "green cursor -- current position"
            n1001 = local read "temperature points"() -> (w2155:dbl[])
            n1002 = local read "time points"() -> (w2153:dbl[])
            n1003 = call "replace cursor - plot ref.vi"("action"=w2156, "cursor index"=w2147, "Plot ref in"=w2149) -> ("read X"=w2152:dbl, "Plot ref out"=w2148:refnum<vi>)  [unwired: 6 in, 1 out]
            n1004 = Threshold 1D Array(2:w2152, 3:w2153) -> (0:w2151:dbl)  [unwired: 1 in]
            n1005 = Index Array(array=w2155, index=w2151) -> (element=w2146:dbl)
            n1006 = local write "temperature(K)"(w2146) -> ()
            n1007 = call "replace cursor - plot ref.vi"("label"=w2150, "action"=w2154, "cursor index"=w2147, "new  Y"=w2146, "Plot ref in"=w2148) -> ()  [unwired: 4 in, 3 out]
            n1008 = local write "time (min)"(w2152) -> ()
          }
          frame 1..3 {
            # "triple cursor -- bounds"
            n1009 = call "cursor window logic V2.vi"("CursIdx"=w2159, "cursor window action"=cursor_window_action."cursor moves", "cursor window in"=w2158) -> ()  [unwired: 7 in, 2 out]
          }
        }
      }
      event Mouse Enter {
        n1010 = event-data() -> ()  [unwired: 1 in, 1 out]
